vi "1B_ArbTriggeredOn.vi"(5 "Frequency (Hz)":dbl=40000.0, 7 "Amplitude (Vpp)":dbl=3.2, 11 "error in":errorcluster) -> (15 "error out":errorcluster)   [LabVIEW 2010]
uses:
  <instrlib>/Agilent 33XXX Series/Agilent 33XXX Series.lvlib
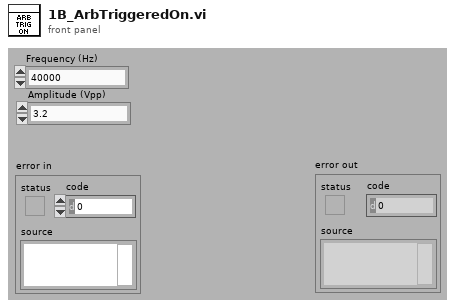
[diagram p1: front panel]
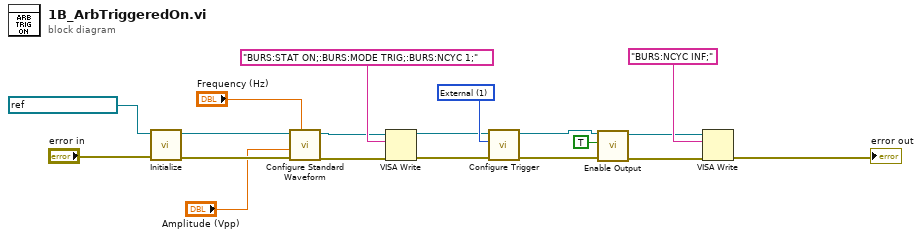
[diagram p0: block diagram]
diagram:
  w16 = u16 1 items=["Internal", "External", "Software (bus)"] ("Trigger Source (0: Internal)")
  n1 = call <instrlib>:"Initialize.vi"("error in (no error)"="error in", "VISA resource name"=refnum<visa-resource-name> "GPIB0::7::INSTR") -> ("error out"=w18:errorcluster, "VISA resource name out"=w17:refnum<visa-resource-name>)  [unwired: 8 in]
  n2 = call <instrlib>:"Configure Standard Waveform.vi"("Frequency (1000 Hz)"="Frequency (Hz)", "error in (no error)"=w18, "Amplitude (1)"="Amplitude (Vpp)", "VISA resource name"=w17) -> ("error out"=w11:errorcluster, "VISA resource name out"=w12:refnum<visa-resource-name>)  [unwired: 6 in]
  n3 = VISA Write(VISA resource name=w12, write buffer="BURS:STAT ON;:BURS:MODE TRIG;:BURS:NCYC 1;", error in (no error)=w11) -> (VISA resource name out=w15:refnum<visa-resource-name>, error out=w14:errorcluster)  [unwired: 1 out]
  n4 = call <instrlib>:"Configure Trigger.vi"("error in (no error)"=w14, "Trigger Source (0: Internal)"=w16, "VISA resource name"=w15) -> ("error out"=w7:errorcluster, "VISA resource name out"=w8:refnum<visa-resource-name>)  [unwired: 7 in]
  n5 = call <instrlib>:"Enable Output.vi"("error in (no error)"=w7, "Enable Output  (T: Enable)"=TRUE, "VISA resource name"=w8) -> ("error out"=w5:errorcluster, "VISA resource name out"=w6:refnum<visa-resource-name>)  [unwired: 7 in]
  n6 = VISA Write(VISA resource name=w6, write buffer="BURS:NCYC INF;", error in (no error)=w5) -> (error out=→"error out":errorcluster)  [unwired: 2 out]
